vi "LabVIEW UI Main.vi"() -> ()   [LabVIEW 2017]
uses:
  <vilib>/NI Veristand/Execution/Alarm/AlarmInfo.ctl
  <vilib>/NI Veristand/Execution/Workspace/NodeInfo.ctl
  <vilib>/NI Veristand/Execution/Workspace/Waveform Data Type.ctl
  subVIs/State Enum.ctl
  subVIs/State.ctl
  <vilib>/NI Veristand/Execution/AlarmManager/AlarmManagerAPI.ctl
  <vilib>/NI Veristand/Execution/Workspace/WorkspaceAPI.ctl
  <vilib>/NI Veristand/Execution/Project/Project Ref.ctl
  <vilib>/NI Veristand/Execution/Workspace/NI VeriStand - Get Multiple Channel Values.vi
  <vilib>/NI Veristand/Execution/Workspace/NI_VS Workspace ExecutionAPI.lvlib
  <vilib>/NI Veristand/Execution/AlarmManager/NI_VS AlarmManager ExecutionAPI.lvlib
  NationalInstruments.VeriStand.ClientAPI
  <vilib>/NI Veristand/Execution/Project/NI_VS Project ExecutionAPI.lvlib
  <vilib>/NI Veristand/Execution/Alarm/NI_VS Alarm ExecutionAPI.lvlib
panel:
  out "AI5":dbl caption="T0"
  in  "Project File Path":path
  out "Enum":T1
  in  "Tab Control 2":enum32{"Page 1", "Page 2"}(tab)
  out "AI1":dbl
  out "AI3":dbl
  in  "Restart":bool
  out "Channels":T2[](array[typedef])
  in  "Stop":bool
  out "error out":errorcluster
  out "AI2":dbl caption="T0"
  in  "error in":errorcluster
  out "Alarms Data":T4[](array[typedef]) {"Trip Value" format="%.2f"; "Delay" format="%.2f"; "Low Limit" format="%.2f"; "High Limit" format="%.2f"}
  out "Thermometer":dbl(slide) scale=0.0..100.0
  out "Waveform Chart":dbl[][](graph)
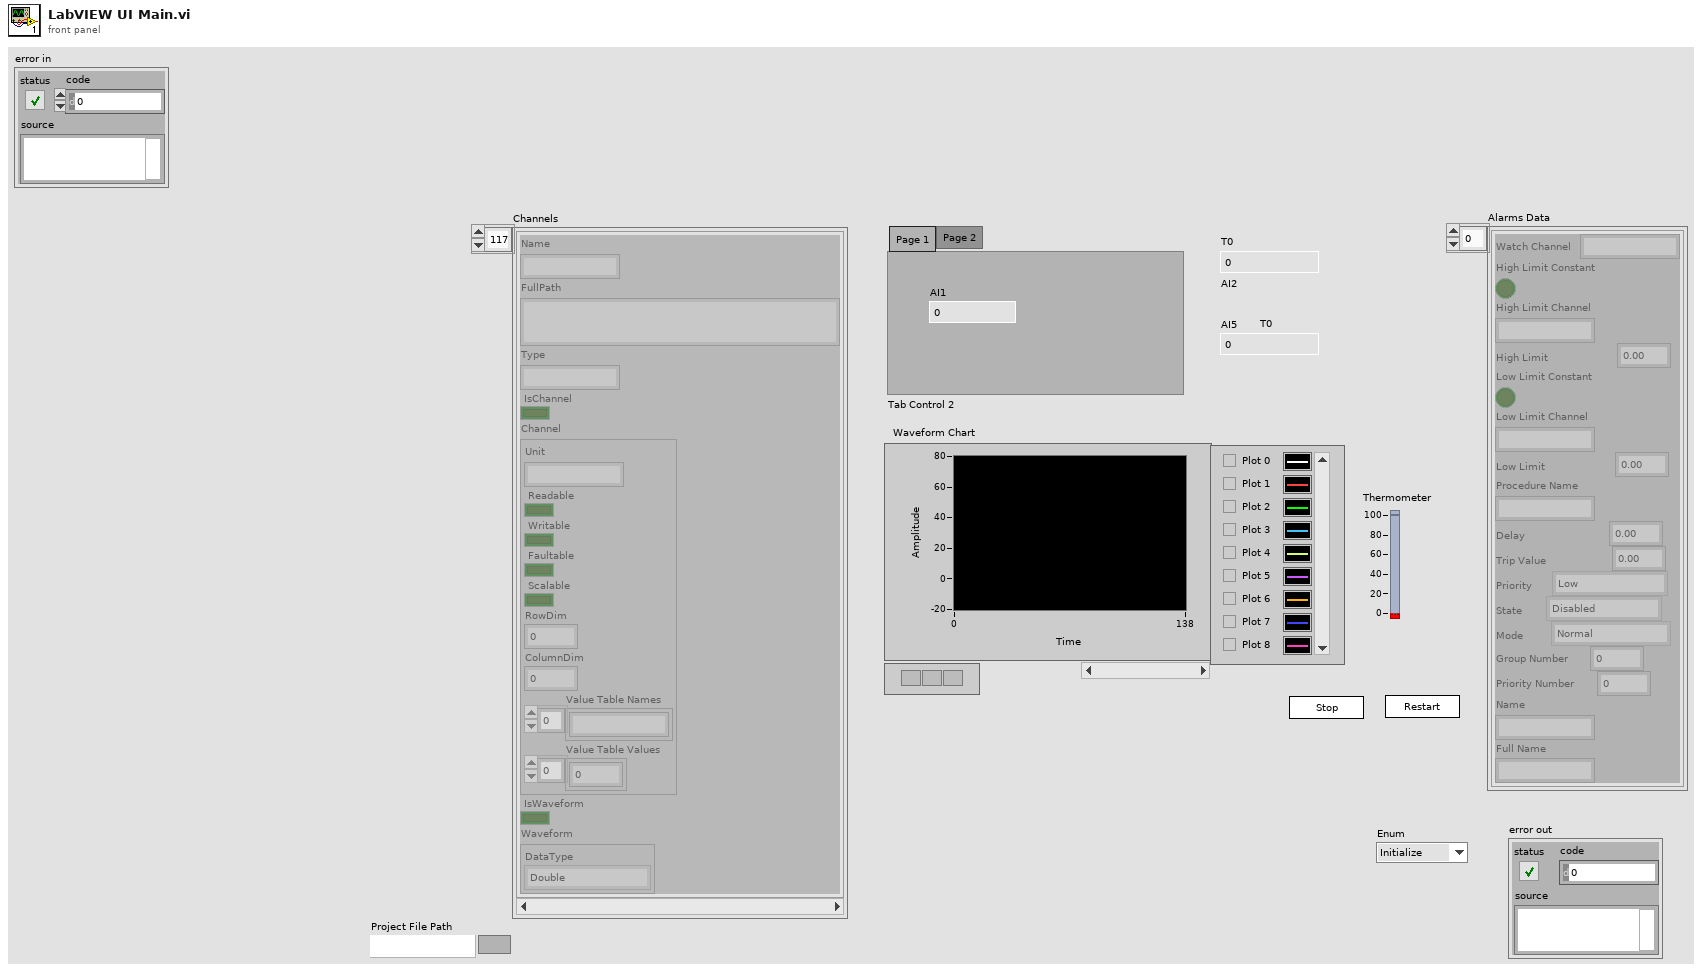
[diagram p1: front panel]
types:
  T1 = typedef "State Enum.ctl" = enum16{"Initialize", "Aquire", "Close"}
  T2 = typedef "NI_VS Workspace ExecutionAPI.lvlib/NodeInfo.ctl" = cluster{"Name":string, "FullPath":string, "Type":string, "IsChannel":bool, "Channel":cluster{"Unit":string, "Readable":bool, "Writable":bool, "Faultable":bool, "Scalable":bool, "RowDim":u32, "ColumnDim":u32, "Value Table Names":string[], "Value Table Values":dbl[]}, "IsWaveform":bool, "Waveform":cluster{"DataType":T3}}
  T3 = typedef "NI_VS Workspace ExecutionAPI.lvlib/Waveform Data Type.ctl" = enum16{"Double", "ComplexDouble"}
  T4 = typedef "NI_VS Alarm ExecutionAPI.lvlib/AlarmInfo.ctl" = cluster{"Watch Channel":string, "High Limit Constant":bool, "High Limit Channel":string, "High Limit":dbl, "Low Limit Constant":bool, "Low Limit Channel":string, "Low Limit":dbl, "Procedure Name":string, "Delay":dbl, "Trip Value":dbl, "Priority":enum16{"Low", "Medium", "High"}, "State":enum16{"Disabled", "Enabled", "Tripped", "Delayed Trip", "Indicate"}, "Mode":enum16{"Normal", "Indicate Only"}, "Group Number":u32, "Priority Number":u32, "Name":string, "Full Name":string}
  T5 = typedef "State.ctl" = cluster{"AlarmManager":T6, "WorkspaceManager":T7, "Project Ref":T8, "Restart":bool, "Alarms":string[], "Channel Name":string[], "Control Index":i32[]}
  T6 = typedef "NI_VS AlarmManager ExecutionAPI.lvlib/AlarmManagerAPI.ctl" = refnum<k24>
  T7 = typedef "NI_VS Workspace ExecutionAPI.lvlib/WorkspaceAPI.ctl" = refnum<k24>
  T8 = typedef "NI_VS Project ExecutionAPI.lvlib/Project Ref.ctl" = refnum<k24>
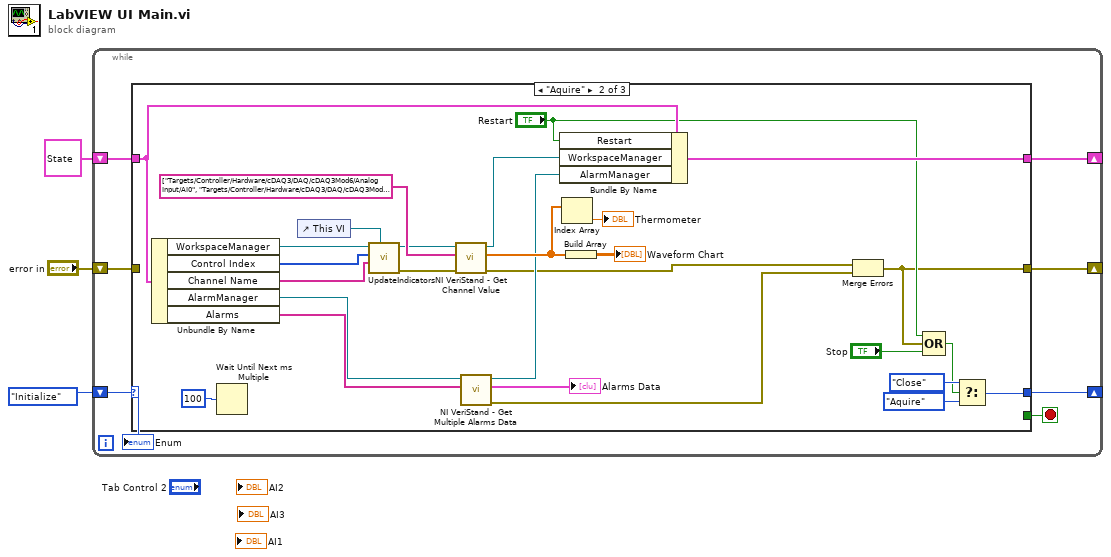
[diagram p0: block diagram]
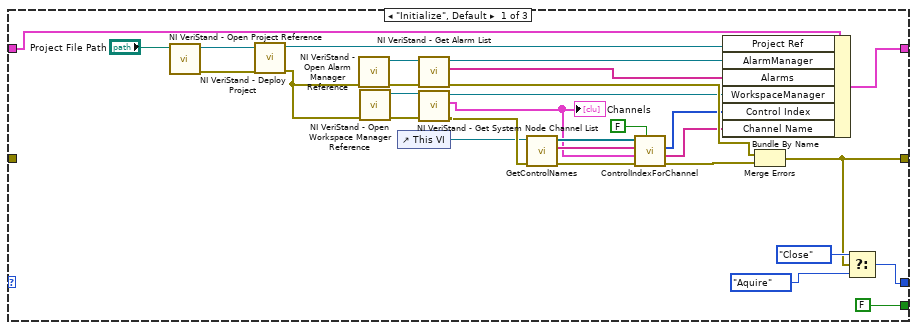
[diagram p2: hidden frame]
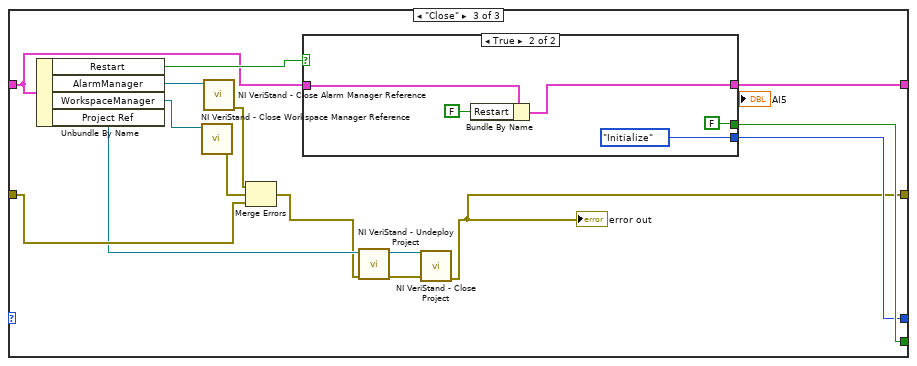
[diagram p3: hidden frame]
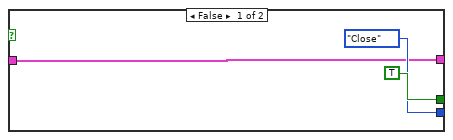
[diagram p4: hidden frame]
diagram:
  n1 = while {
    shift-right: [w4] -> _
    shift-left: State_Enum."Initialize" -> [w10]
    shift-right: [w8] -> _
    shift-left: T5 {"AlarmManager"=refnum, "WorkspaceManager"=refnum, "Project Ref"=refnum, "Restart"=FALSE, "Alarms"=[], "Channel Name"=[], "Control Index"=[]} -> [w9]
    shift-right: [w7] -> _
    shift-left: "error in" -> [w6]
    stop <- w5 stop-if-true
    n2 = case shown="\"Aquire\"" w10 {
      tunnel: [w21 w66 w75] -> w4
      tunnel: w9 -> [w40 w52 w73]
      tunnel: [w39 w51 w74] -> w8
      tunnel: [w19 w42 w68] -> w7
      tunnel: w6 -> [_ _ w76]
      tunnel: [FALSE _ w81] -> w5
      frame "Initialize", Default {
        n3 = call <vilib>:"NI VeriStand - Open Project Reference.vi"("Project File Path"="Project File Path") -> ("error out"=w14:errorcluster, "Project Ref"=w16:T8)  [unwired: 9 in]
        n4 = call <vilib>:"NI VeriStand - Deploy Project.vi"("error in (no error)"=w14, "Project Ref in"=w16) -> ("error out"=w13:errorcluster, "Project Ref out"=w15:T8)  [unwired: 8 in]
        n5 = call <vilib>:"NI VeriStand - Open Alarm Manager Reference.vi"("error in (no error)"=w13) -> ("error out"=w37:errorcluster, "AlarmManager"=w38:T6)  [unwired: 9 in]
        n6 = call <vilib>:"NI VeriStand - Open Workspace Manager Reference.vi"("error in (no error)"=w13) -> ("error out"=w33:errorcluster, "WorkspaceManager"=w11:T7)  [unwired: 9 in]
        n7 = control-ref of="This VI"() -> (w18:refnum<vi>)
        n8 = call <vilib>:"NI VeriStand - Get Alarm List.vi"("error in (no error)"=w37, "AlarmManager in"=w38) -> ("error out"=w36:errorcluster, "alarms"=w35:string[], "AlarmManager out"=w34:T6)  [unwired: 7 in]
        n9 = call <vilib>:"NI VeriStand - Get System Node Channel List.vi"("error in (no error)"=w33, "WorkspaceManager in"=w11) -> ("error out"=w29:errorcluster, "Channels"=w30:T2[], "WorkspaceManager out"=w26:T7)  [unwired: 7 in]
        "Channels" <- w30
        n10 = call "GetControlNames.vi"("error in (no error)"=w29, "VI in"=w18) -> ("error out"=w28:errorcluster, "Array 2"=w32:string[], "Array"=w31:refnum<vi>[])  [unwired: 7 in]
        n11 = call "ControlIndexForChannel.vi"("Full Path"=FALSE, "error in (no error)"=w28, "Versitand Channels"=w30, "Control Names"=w32, "Controls References"=w31) -> ("error out"=w27:errorcluster, "Channel Name"=w24:string[], "Control Index"=w25:i32[])  [unwired: 4 in]
        n12 = Bundle By Name(cluster=w40, "Project Ref"=w15, "AlarmManager"=w34, "Alarms"=w35, "WorkspaceManager"=w26, "Control Index"=w25, "Channel Name"=w24) -> (w39:T5)
        n13 = Merge Errors(w36, w27) -> (w19:errorcluster)
        n14 = Select(t=State_Enum."Close", s=w19, f=State_Enum."Aquire" ("Enum")) -> (s? t:f=w21:T1)
      }
      frame "Aquire" {
        n15 = Unbundle By Name(w52) -> ("WorkspaceManager"=w55:T7, "Control Index"=w54:i32[], "Channel Name"=w53:string[], "AlarmManager"=w49:T6, "Alarms"=w48:string[])
        n16 = Wait Until Next ms Multiple(millisecond multiple=u32 100) -> ()  [unwired: 1 out]
        n17 = control-ref of="This VI"() -> (w56:refnum<vi>)
        n18 = call "UpdateIndicators.vi"("VI in"=w56, "Channel Name"=w53, "Control Index"=w54, "WorkspaceManager in"=w55) -> ("error out"=w60:errorcluster, ".NET Refnum out"=w59:T7)  [unwired: 6 in]
        n19 = call-poly <vilib>:"NI VeriStand - Get Channel Value.vi"("error in (no error)"=w60, "Channels"=string[] ["Targets/Controller/Hardware/cDAQ3/DAQ/cDAQ3Mod6/Analog Input/AI0", "Targets/Controller/Hardware/cDAQ3/DAQ/cDAQ3Mod6/Analog Input/AI5", "Targets/Controller/Hardware/cDAQ3/DAQ/cDAQ3Mod6/Analog Input/AI2"] ("Channels 2"), "WorkspaceManager in"=w59) -> ("error out"=w46:errorcluster, "Values"=w62:dbl[], "WorkspaceManager out"=w50:T7)  [unwired: 6 in]
        n20 = call <vilib>:"NI VeriStand - Get Multiple Alarms Data.vi"("Alarm Names"=w48, "AlarmManager in"=w49) -> ("error out"=w45:errorcluster, "Alarms Data"=→"Alarms Data":T4[], "AlarmManager out"=w47:T6)  [unwired: 7 in]
        n21 = Bundle By Name(cluster=w52, "Restart"="Restart", "WorkspaceManager"=w50, "AlarmManager"=w47) -> (w51:T5)
        n22 = Index Array(array=w62) -> (element=→"Thermometer":dbl)  [unwired: 1 in]
        n23 = Build Array(w62) -> (→"Waveform Chart":dbl[][])
        n24 = Merge Errors(w46, w45) -> (w42:errorcluster)
        n25 = Compound Arithmetic op=OR("Restart", w42, "Stop") -> (w44:bool)
        n26 = Select(t=State_Enum."Close", s=w44, f=State_Enum."Aquire" ("Enum")) -> (s? t:f=w66:T1)
      }
      frame "Close" {
        n27 = Unbundle By Name(w73) -> ("Restart"=w82:bool, "AlarmManager"=w79:T6, "WorkspaceManager"=w80:T7, "Project Ref"=w72:T8)
        n28 = call <vilib>:"NI VeriStand - Close Workspace Manager Reference.vi"("WorkspaceManager"=w80) -> ("error out"=w77:errorcluster)  [unwired: 10 in]
        n29 = call <vilib>:"NI VeriStand - Close Alarm Manager Reference.vi"("AlarmManager"=w79) -> ("error out"=w78:errorcluster)  [unwired: 10 in]
        n30 = Merge Errors(w78, w77, w76) -> (w69:errorcluster)
        n31 = case shown="True" w82 {
          tunnel: [TRUE FALSE] -> w81
          tunnel: [State_Enum."Close" ("Enum") State_Enum."Initialize" ("Enum")] -> w75
          tunnel: [w83 w86] -> w74
          tunnel: w73 -> [w83 w88]
          frame False {
          }
          frame True {
            n32 = Bundle By Name(cluster=w88, "Restart"=FALSE) -> (w86:T5)
          }
        }
        n33 = call <vilib>:"NI VeriStand - Undeploy Project.vi"("error in (no error)"=w69, "Project Ref in"=w72) -> ("error out"=w70:errorcluster, "Project Ref out"=w71:T8)  [unwired: 8 in]
        n34 = call <vilib>:"NI VeriStand - Close Project.vi"("error in (no error)"=w70, "Project Ref in"=w71) -> ("error out"=w68:errorcluster)  [unwired: 8 in, 1 out]
        "error out" <- w68
      }
    }
    "Enum" <- w10
  }
